vi "Write Path Too Long To Fit.vi"(5 "Path Too Long To Fit":enum32{"Abbreviate Path", "Clip Path"}(ring), 9 "Path in":refnum<class "Path.lvclass">) -> (3 "Path out":refnum<class "Path.lvclass">)   [LabVIEW 2014, in "Path.lvclass"]
uses:
  Path.lvclass
  Path.lvclass/Path.ctl
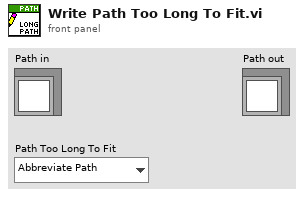
[diagram p1: front panel]
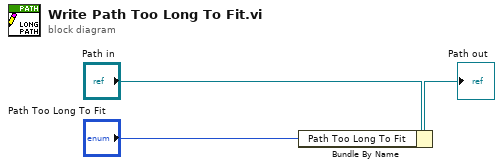
[diagram p0: block diagram]
diagram:
  n1 = Bundle By Name(cluster="Path in", "Path Too Long To Fit"="Path Too Long To Fit") -> (→"Path out":refnum<class "Path.lvclass">)
